vi "Get Current Values and Exec.vi"(3 "Instrument Array":T1[](array[typedef]) {"Private"."Offset" format="%^_3e"; "Private"."Scale Factors" format="%^_3e"}, 4 "Instrument List":i32, 5 "queue in":refnum<queue>) -> (0 "VI Ref":T4, 1 "Valid":bool, 2 "queue out":refnum<queue>)   [LabVIEW 2019]
uses:
  Sub Controls/Instrument Properties.ctl
  Sub Controls/Public.ctl
  Sub Controls/Private.ctl
  Sub Controls/Instrument Ref.ctl
  Sub Controls/SystemCheckBox-resize.ctl
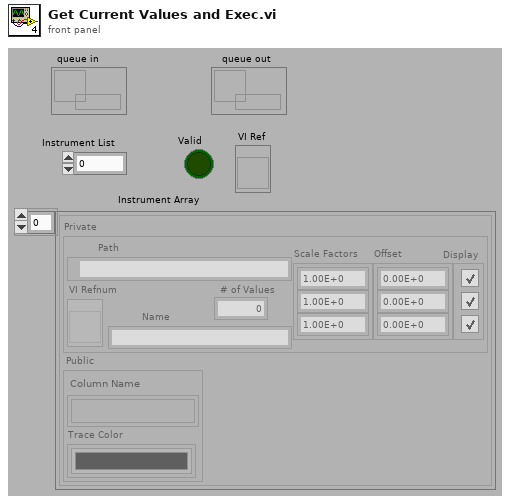
[diagram p1: front panel]
types:
  T1 = typedef "Instrument Properties.ctl" = cluster{"Public":T2, "Private":T3}
  T2 = typedef "Public.ctl" = cluster{"Column Name":string[], "Trace Color":u32[]}
  T3 = typedef "Private.ctl" = cluster{"Path":path, "VI Refnum":T4, "Name":string, "# of Values":i32, "Scale Factors":dbl[], "Display":T5[], "Offset":dbl[]}
  T4 = typedef "Instrument Ref.ctl" = refnum<vi>
  T5 = typedef "SystemCheckBox-resize.ctl" = bool
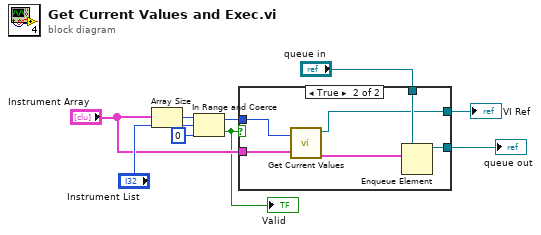
[diagram p0: block diagram]
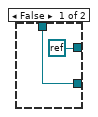
[diagram p2: hidden frame]
diagram:
  n1 = Array Size(array="Instrument Array") -> (size(s)=w9:i32)
  n2 = In Range and Coerce(upper limit=w9, x="Instrument List", lower limit=0) -> (coerced(x)=w5:i32, In Range?=w1:bool)
  "Valid" <- w1
  n3 = case shown="True" w1 {
    tunnel: [w11 w16] -> w2
    tunnel: "queue in" -> [w11 w15]
    tunnel: w5 -> [_ w14]
    tunnel: "Instrument Array" -> [_ w13]
    tunnel: [refnum<k0> refnum w12] -> w3
    frame False {
    }
    frame True {
      n4 = call "Get Current Values.vi"("Instrument List"=w14, "Array"=w13) -> ("VI Ref"=w12:T4, "Instrument"=w17:T1)  [unwired: 2 out]
      n5 = Enqueue Element(queue=w15, element=w17) -> (queue out=w16:refnum<queue>)  [unwired: 2 in, 2 out]
    }
  }
  "queue out" <- w2
  "VI Ref" <- w3
